vi "constant--blank_neighbour_square.vi"() -> (0 "blank_neighbour_square":T1)   [LabVIEW 2020, in "core.lvlib" / "core_data.lvlib"]
uses:
  core_data.lvlib
  neighbour_square.ctl
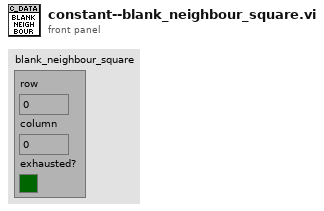
[diagram p1: front panel]
types:
  T1 = typedef "core.lvlib/core_data.lvlib/neighbour_square.ctl" = cluster{"row":u8, "column":u8, "exhausted?":bool}
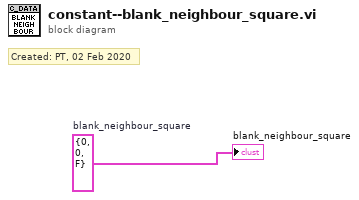
[diagram p0: block diagram]
diagram:
  w1 = T1 {"row"=0, "column"=0, "exhausted?"=FALSE}  # blank_neighbour_square
  # "Created: PT, 02 Feb 2020"
  "blank_neighbour_square" <- w1
